vi "DPT Create Save Directory.vi"(7 "Pass Fail Lab Eval":string, 8 "error in (no error)":errorcluster, 9 "Lab ID":string, 10 "TR Number":string, 11 "FileName DataLog":path) -> (0 "error out":errorcluster, 3 "File Path":path)   [LabVIEW 2016]
panel:
  out "match substring":string
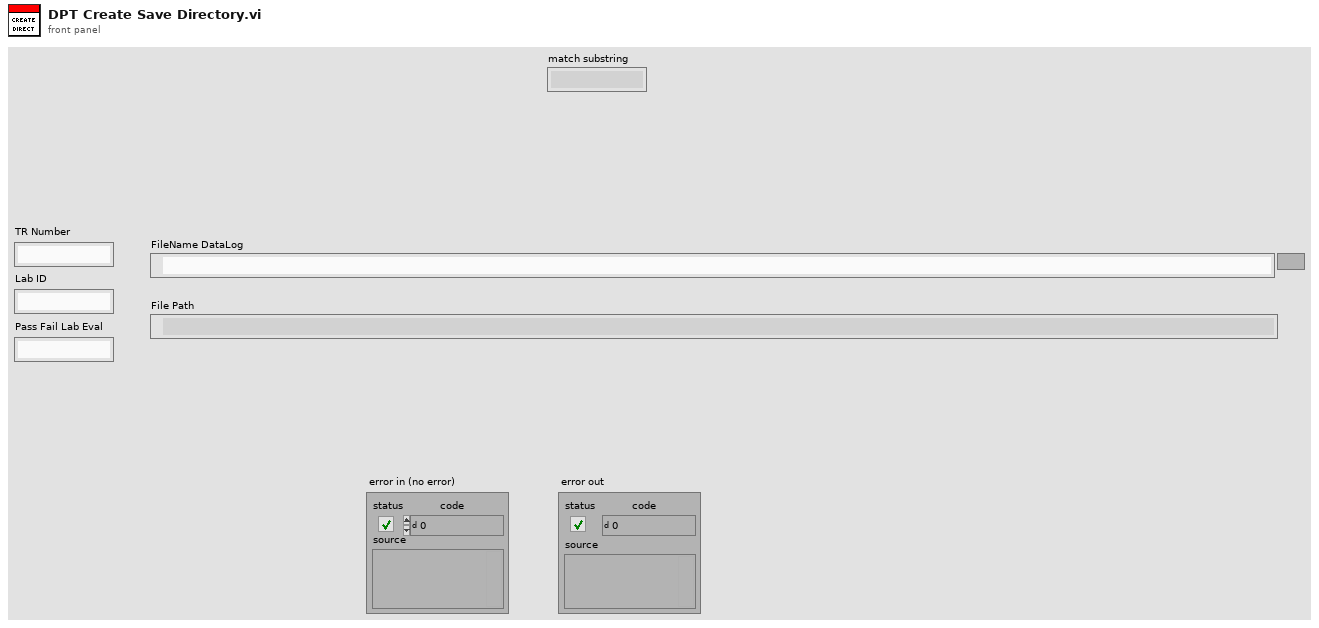
[diagram p1: front panel]
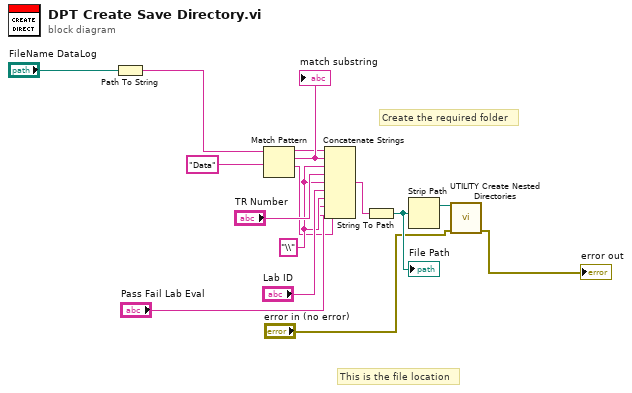
[diagram p0: block diagram]
diagram:
  w5 = "\\"
  # "This is the file location"
  # "Create the required folder"
  n1 = Path To String(path="FileName DataLog") -> (string=w14:string)
  n2 = Match Pattern(string=w14, regular expression="Data") -> (before substring=w9:string, match substring=w12:string, after substring=w3:string)  [unwired: 1 in, 1 out]
  "match substring" <- w12
  n3 = Concatenate Strings(w9, w12, w5, "TR Number", w5, "Lab ID", w5, "Pass Fail Lab Eval", w3) -> (w8:string)
  n4 = String To Path(string=w8) -> (path=w7:path)
  "File Path" <- w7
  n5 = Strip Path(path=w7) -> (stripped path=w6:path)  [unwired: 1 out]
  n6 = call "UTILITY Create Nested Directories.vi"("path to create"=w6, "error in"="error in (no error)") -> ("error out"=→"error out":errorcluster)  [unwired: 11 in, 2 out]
